vi "init Jl server & LV client.vi"(8 "error in (no error)":errorcluster, 9 "Base path (not a path)":path=path "", 11 "Julia user functions script":path) -> (0 "error out":errorcluster, 2 "Jl Server state out":T1, 3 "timeout?":bool)   [LabVIEW 2018, in "LV-0mq-Julia_roundtrip-lib.lvlib" / "LV2Julia_core.lvlib"]
doc: "Init Julia server & LabView client."
uses:
  LV2Julia_core.lvlib
  Server or client state.ctl
  Commands.ctl
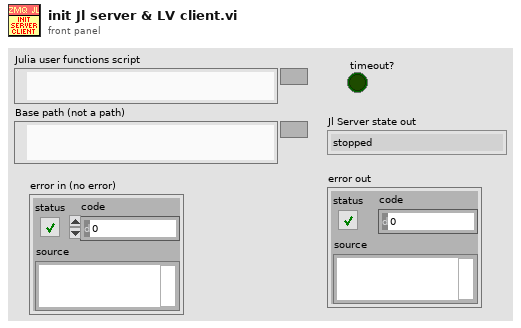
[diagram p1: front panel]
types:
  T1 = typedef "LV-0mq-Julia_roundtrip-lib.lvlib/LV2Julia_core.lvlib/Server or client state.ctl" = enum16{"stopped", "running", "unknown"}
  T2 = typedef "LV-0mq-Julia_roundtrip-lib.lvlib/LV2Julia_core.lvlib/Commands.ctl" = enum16{"Start Jl-server & Init LV-client", "Send request & Get response ", "Stop Jl-server & Cleanup LV-client", "Cleanup LV-client", "Start Jl-server", "Stop Jl-server", "Init LV-Client", "Cleanup LV-Client", "(not allowed)", "Set LV Client state", "Set Jl Server state", "set ZMQ timeout", "read ZMQ timeout", "read-out state"}
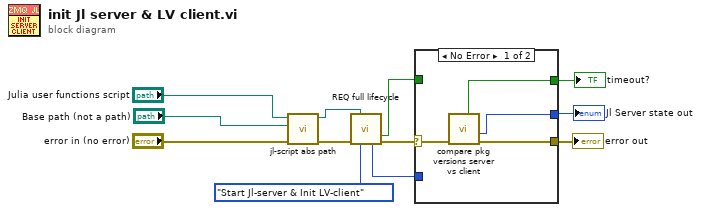
[diagram p0: block diagram]
diagram:
  n1 = call "jl-script abs path.vi"("error in (no error)"="error in (no error)", "Base path (not a path)"="Base path (not a path)", "Julia user functions script"="Julia user functions script") -> ("error out"=w4:errorcluster, "script abs path"=w3:path)  [unwired: 7 in]
  n2 = call "REQ full lifecycle.vi"("Julia user functions script"=w3, "error in"=w4, "command"=Commands."Start Jl-server & Init LV-client") -> ("timeout?"=w8:bool, "Jl Server state out"=w11:T1, "error out"=w7:errorcluster)  [unwired: 6 in, 4 out]
  n3 = case shown="No Error" w7 {
    selector: w7 -> [w16 w18]
    tunnel: [w14 w19] -> w9
    tunnel: w8 -> [_ w19]
    tunnel: [w15 w18] -> w10
    tunnel: [w13 w17] -> w12
    tunnel: w11 -> [_ w17]
    frame No Error {
      n4 = call "compare pkg versions server vs client.vi"("error in (no error)"=w16) -> ("error out"=w15:errorcluster, "Jl Server state out"=w13:T1, "timeout?"=w14:bool)  [unwired: 4 in, 4 out]
    }
    frame Error {
    }
  }
  "Jl Server state out" <- w12
  "error out" <- w10
  "timeout?" <- w9
